vi "Teleop.vi"(10 "Match Info":T1={"Autonomous Elapsed Seconds"=0.0, "TeleOp Elapsed Seconds"=0.0, "Disabled Elapsed Seconds"=0.0, "Visited Autonomous"=FALSE, "Visited TeleOp"=FALSE, "Visited Disabled"=FALSE, "Autonomous Settings"={"Autonomous Style"=enum."Independent", "VI Refnum"=refnum}}, 11 "Call Context":T2) -> ()   [LabVIEW 2013]
doc: "This VI is called for each TeleOp packet received from the DS where the robot is not disabled. It is often used to read from the joysticks and update I/O or to update setpoints for timed control loops. It should complete and return within 20 milliseconds or it may miss DS packets."
uses:
  <vilib>/Rock Robotics/WPI/DriverStation/WPI_DriverStationDerivedRobotMode.ctl
  <vilib>/Rock Robotics/WPI/DriverStation/WPI_DriverStationMatch Info.ctl
  Robot Global Data.vi
  <vilib>/Rock Robotics/WPI/Joystick/WPI_JoystickGetSetRefNum.vi
panel:
  in  "Left":bool
  in  "Right":bool
  in  "Shifter":bool
  in  "HarvSpeed":dbl=0.5
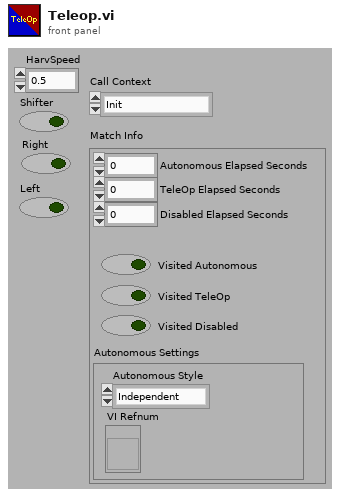
[diagram p1: front panel]
types:
  T1 = typedef "WPI_DriverStationMatch Info.ctl" = cluster{"Autonomous Elapsed Seconds":dbl, "TeleOp Elapsed Seconds":dbl, "Disabled Elapsed Seconds":dbl, "Visited Autonomous":bool, "Visited TeleOp":bool, "Visited Disabled":bool, "Autonomous Settings":cluster{"Autonomous Style":enum16{"Iterative", "Independent"}, "VI Refnum":refnum<vi>}}
  T2 = typedef "WPI_DriverStationDerivedRobotMode.ctl" = enum16{"Init", "Execute", "Stop"}
  T3 = typedef "WPI_JoystickDevRef.ctl" = cluster{"Device":T4}
  T4 = typedef "WPI_JoystickDeviceEnum.ctl" = enum16{"USB 1", "USB 2", "USB 3", "USB 4", "Kinect 1", "Kinect 2"}
  T5 = cluster{"axis 1 (x)":dbl, "axis 2 (y)":dbl, "axis 3 (throttle)":dbl, "axis 4":dbl, "axis 5":dbl, "axis 6":dbl}
  T6 = typedef "WPI_MotorControlDeviceRef.ctl" = cluster{"DeviceStatus":errorcluster, "Type":enum16{"PWM", "CAN"}, "PWM":cluster{"Digital Module":T7, "PWM Channel":T8, "DeadBand":T9}, "CAN":cluster{"Device Number":u8, "Control Mode":T10, "Semaphore":T11, "Max Vout":dbl}, "Invert":bool, "TransformRef":T12, "InvTransformRef":T12}
  T7 = typedef "FPGA_TypedefDigitalModule.ctl" = enum16{"Digital Module 1", "Digital Module 2"}
  T8 = typedef "FPGA_DIOPWMChannel.ctl" = enum8{"PWM 1", "PWM 2", "PWM 3", "PWM 4", "PWM 5", "PWM 6", "PWM 7", "PWM 8", "PWM 9", "PWM 10", "Invalid"}
  T9 = typedef "WPI_PWMDeadband.ctl" = cluster{"Name":string, "maxPositivePwm":i32, "minPositivePwm":i32, "centerPwm":i32, "maxNegativePwm":i32, "minNegativePwm":i32, "angularRange":u16}
  T10 = typedef "WPI_CANJaguar_ControlMode.ctl" = enum8{"Percent VBus", "Current", "Speed", "Position", "Voltage"}
  T11 = typedef "Semaphore RefNum" = refnum<k1>
  T12 = typedef "WPI_PWMTransform_ConPane.ctl" = refnum<vi>
  T13 = cluster{"RightLow":dbl, "LeftLow":dbl, "RightHigh":dbl, "LeftHigh":dbl}
  T14 = cluster{"Driver Station Digital Input (1-8)[0]":bool, "Driver Station Digital Input (1-8)[1]":bool, "Driver Station Digital Input (1-8)[2]":bool, "Driver Station Digital Input (1-8)[3]":bool, "Driver Station Digital Input (1-8)[4]":bool, "Driver Station Digital Input (1-8)[5]":bool, "Driver Station Digital Input (1-8)[6]":bool, "Driver Station Digital Input (1-8)[7]":bool, "Driver Station Digital Input (1-8)[8]":bool}
  T15 = typedef "WPI_JoystickButtonState.ctl" = cluster{"Button 1":bool, "Button 2":bool, "Button 3":bool, "Button 4":bool, "Button 5":bool, "Button 6":bool, "Button 7":bool, "Button 8":bool, "Button 9":bool, "Button 10":bool, "Button 11":bool, "Button 12":bool}
  T16 = typedef "WPI_ServoDeviceRef.ctl" = cluster{"DeviceStatus":errorcluster, "Digital Module":T7, "PWM Channel":T8, "DeadBand":T9}
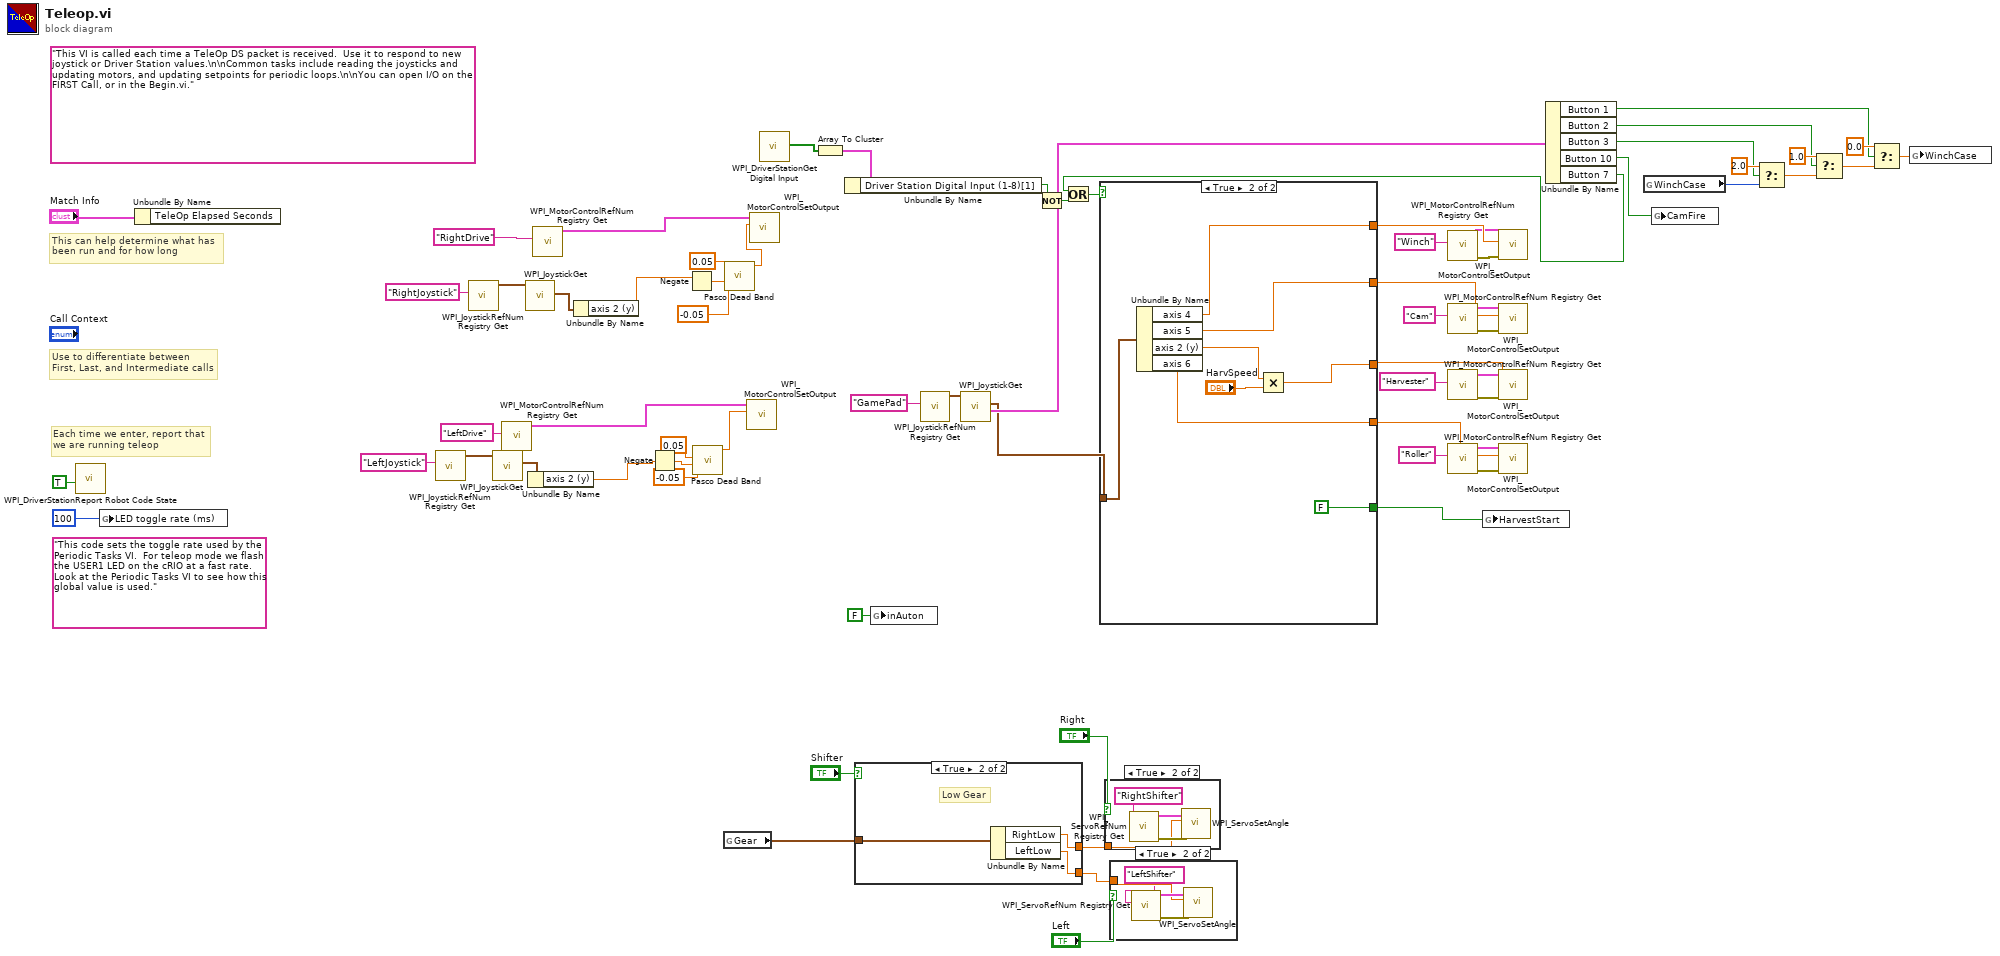
[diagram p0: block diagram]
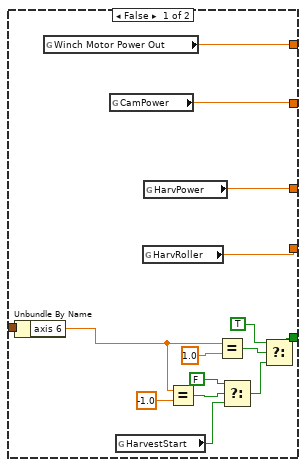
[diagram p2: hidden frame]
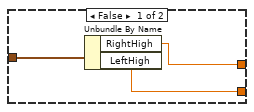
[diagram p4: hidden frame]
diagram:
  (unwired) "This code sets the toggle rate used by the Periodic Tasks VI.  For teleop mode we flash the USER1 LED on the cRIO at a fast rate.  Look at the Periodic Tasks VI to see how this global value is used."
  (unwired) "This VI is called each time a TeleOp DS packet is received.  Use it to respond to new joystick or Driver Station values.\n\nCommon tasks include reading the joysticks and updating motors, and updating setpoints for periodic loops.\n\nYou can open I/O on the FIRST Call, or in the Begin.vi."
  # "Each time we enter, report that\nwe are running teleop"
  # "Use to differentiate between\nFirst, Last, and Intermediate calls"
  # "This can help determine what has\nbeen run and for how long"
  n1 = call <vilib>:"WPI_DriverStationReport Robot Code State.vi"("TeleOp"=TRUE ("Autonomous")) -> ()  [unwired: 10 in, 1 out]
  n2 = global write "Robot Global Data.vi" "LED toggle rate (ms)"(u32 100 ("LED ms toggle rate")) -> ()
  n3 = Unbundle By Name("Match Info") -> ()  [unwired: 1 out]
  n4 = call <vilib>:"WPI_JoystickRefNum Registry Get.vi"("refnum name"="LeftJoystick") -> ("JoystickDevRef"=w57:T3)  [unwired: 9 in, 1 out]
  n5 = call <vilib>:"WPI_JoystickRefNum Registry Get.vi"("refnum name"="RightJoystick") -> ("JoystickDevRef"=w62:T3)  [unwired: 9 in, 1 out]
  n6 = call <vilib>:"WPI_JoystickGet.vi"("JoystickDevRef"=w57) -> ("Axes"=w56:T5)  [unwired: 4 in, 2 out]
  n7 = call <vilib>:"WPI_MotorControlRefNum Registry Get.vi"("refnum name"="LeftDrive") -> ("MotorControlDevRef"=w60:T6)  [unwired: 9 in, 1 out]
  n8 = call <vilib>:"WPI_JoystickGet.vi"("JoystickDevRef"=w62) -> ("Axes"=w61:T5)  [unwired: 4 in, 2 out]
  n9 = Unbundle By Name(w56) -> ("axis 2 (y)"=w55:dbl)
  n10 = call <vilib>:"WPI_MotorControlRefNum Registry Get.vi"("refnum name"="RightDrive") -> ("MotorControlDevRef"=w65:T6)  [unwired: 9 in, 1 out]
  n11 = Unbundle By Name(w61) -> ("axis 2 (y)"=w54:dbl)
  n12 = Negate(x=w55) -> (-x=w49:dbl)
  n13 = Negate(x=w54) -> (-x=w53:dbl)
  n14 = call "Pasco Dead Band.vi"("lower limit"=-0.05, "PWM Power"=w49, "upper limit"=0.05) -> ("PWM Power"=w46:dbl)  [unwired: 7 in, 1 out]
  n15 = global read "Robot Global Data.vi" "Gear"() -> (w45:T13)
  n16 = call "Pasco Dead Band.vi"("lower limit"=-0.05, "PWM Power"=w53, "upper limit"=0.05) -> ("PWM Power"=w52:dbl)  [unwired: 7 in, 1 out]
  n17 = call <vilib>:"WPI_MotorControlSetOutput.vi"("Output"=w46, "MotorControlDevRef"=w60) -> ()  [unwired: 7 in, 3 out]
  n18 = call <vilib>:"WPI_MotorControlSetOutput.vi"("Output"=w52, "MotorControlDevRef"=w65) -> ()  [unwired: 7 in, 3 out]
  n19 = call <vilib>:"WPI_DriverStationGet Digital Input.vi"() -> ("Driver Station Digital Input (1-8)"=w5:bool[])  [unwired: 11 in]
  n20 = Array To Cluster(array=w5) -> (cluster=w4:T14)
  n21 = Unbundle By Name(w4) -> ("Driver Station Digital Input (1-8)[1]"=w3:bool)
  n22 = case shown="True" "Shifter" {
    tunnel: w45 -> [w71 w74]
    tunnel: [w70 w73] -> w44
    tunnel: [w69 w72] -> w43
    frame False {
      n23 = Unbundle By Name(w71) -> ("RightHigh"=w70:dbl, "LeftHigh"=w69:dbl)
    }
    frame True {
      # "Low Gear"
      n24 = Unbundle By Name(w74) -> ("RightLow"=w73:dbl, "LeftLow"=w72:dbl)
    }
  }
  n25 = global write "Robot Global Data.vi" "inAuton"(FALSE ("inAuton")) -> ()
  n26 = call <vilib>:"WPI_JoystickRefNum Registry Get.vi"("refnum name"="GamePad") -> ("JoystickDevRef"=w38:T3)  [unwired: 9 in, 1 out]
  n27 = call <vilib>:"WPI_JoystickGet.vi"("JoystickDevRef"=w38) -> ("Buttons"=w11:T15, "Axes"=w9:T5)  [unwired: 4 in, 1 out]
  n28 = Not(x=w3) -> (.not. x?=w2:bool)
  n29 = case shown="True" "Right" {
    tunnel: w44 -> [_ w75]
    frame False {
    }
    frame True {
      n30 = call <vilib>:"WPI_ServoRefNum Registry Get.vi"("refnum name"="RightShifter") -> ("error out"=w78:errorcluster, "ServoDeviceRef"=w77:T16)  [unwired: 9 in]
      n31 = call <vilib>:"WPI_ServoSetAngle.vi"("error in (no error)"=w78, "Angle"=w75, "ServoDeviceRef"=w77) -> ()  [unwired: 7 in, 2 out]
    }
  }
  n32 = case shown="True" "Left" {
    tunnel: w43 -> [_ w80]
    frame False {
    }
    frame True {
      n33 = call <vilib>:"WPI_ServoRefNum Registry Get.vi"("refnum name"="LeftShifter") -> ("error out"=w81:errorcluster, "ServoDeviceRef"=w82:T16)  [unwired: 9 in]
      n34 = call <vilib>:"WPI_ServoSetAngle.vi"("error in (no error)"=w81, "Angle"=w80, "ServoDeviceRef"=w82) -> ()  [unwired: 7 in, 2 out]
    }
  }
  n35 = call <vilib>:"WPI_MotorControlRefNum Registry Get.vi"("refnum name"="Winch") -> ("error out"=w29:errorcluster, "MotorControlDevRef"=w23:T6)  [unwired: 9 in]
  n36 = call <vilib>:"WPI_MotorControlRefNum Registry Get.vi"("refnum name"="Cam") -> ("error out"=w28:errorcluster, "MotorControlDevRef"=w27:T6)  [unwired: 9 in]
  n37 = call <vilib>:"WPI_MotorControlRefNum Registry Get.vi"("refnum name"="Harvester") -> ("error out"=w33:errorcluster, "MotorControlDevRef"=w32:T6)  [unwired: 9 in]
  n38 = call <vilib>:"WPI_MotorControlRefNum Registry Get.vi"("refnum name"="Roller") -> ("error out"=w35:errorcluster, "MotorControlDevRef"=w36:T6)  [unwired: 9 in]
  n39 = Unbundle By Name(w11) -> ("Button 1"=w14:bool, "Button 2"=w15:bool, "Button 3"=w16:bool, "Button 10"=w10:bool, "Button 7"=w6:bool)
  n40 = Or(x=w6, y=w2) -> (x .or. y?=w7:bool)
  n41 = case shown="True" w7 {
    tunnel: [w97 w104] -> w34
    tunnel: [w96 w99] -> w30
    tunnel: w9 -> [w84 w105]
    tunnel: [w94 w103] -> w24
    tunnel: [w95 w102] -> w22
    tunnel: [w83 FALSE ("HarvestStart")] -> w8
    frame False {
      n42 = Unbundle By Name(w84) -> ("axis 6"=w92:dbl)
      n43 = global read "Robot Global Data.vi" "Winch Motor Power Out"() -> (w94:dbl)
      n44 = global read "Robot Global Data.vi" "CamPower"() -> (w95:dbl)
      n45 = global read "Robot Global Data.vi" "HarvestStart"() -> (w93:bool)
      n46 = global read "Robot Global Data.vi" "HarvRoller"() -> (w97:dbl)
      n47 = global read "Robot Global Data.vi" "HarvPower"() -> (w96:dbl)
      n48 = Equal?(x=w92, y=-1.0) -> (x = y?=w91:bool)
      n49 = Equal?(x=w92, y=1.0) -> (x = y?=w86:bool)
      n50 = Select(t=FALSE, s=w91, f=w93) -> (s? t:f=w89:bool)
      n51 = Select(t=TRUE, s=w86, f=w89) -> (s? t:f=w83:bool)
    }
    frame True {
      n52 = Unbundle By Name(w105) -> ("axis 4"=w103:dbl, "axis 5"=w102:dbl, "axis 2 (y)"=w100:dbl, "axis 6"=w104:dbl)
      n53 = Multiply(x=w100, y="HarvSpeed") -> (x*y=w99:dbl)
    }
  }
  n54 = global write "Robot Global Data.vi" "HarvestStart"(w8) -> ()
  n55 = call <vilib>:"WPI_MotorControlSetOutput.vi"("error in (no error)"=w29, "Output"=w24, "MotorControlDevRef"=w23) -> ()  [unwired: 6 in, 3 out]
  n56 = call <vilib>:"WPI_MotorControlSetOutput.vi"("error in (no error)"=w28, "Output"=w22, "MotorControlDevRef"=w27) -> ()  [unwired: 6 in, 3 out]
  n57 = call <vilib>:"WPI_MotorControlSetOutput.vi"("error in (no error)"=w33, "Output"=w30, "MotorControlDevRef"=w32) -> ()  [unwired: 6 in, 3 out]
  n58 = call <vilib>:"WPI_MotorControlSetOutput.vi"("error in (no error)"=w35, "Output"=w34, "MotorControlDevRef"=w36) -> ()  [unwired: 6 in, 3 out]
  n59 = global read "Robot Global Data.vi" "WinchCase"() -> (w12:i32)
  n60 = global write "Robot Global Data.vi" "CamFire"(w10) -> ()
  n61 = Select(t=2.0, s=w16, f=w12) -> (s? t:f=w21:dbl)
  n62 = Select(t=1.0, s=w15, f=w21) -> (s? t:f=w20:dbl)
  n63 = Select(t=0.0, s=w14, f=w20) -> (s? t:f=w13:dbl)
  n64 = global write "Robot Global Data.vi" "WinchCase"(w13) -> ()
